vi "TagDisplayContainer.vi"(7 "Name(\"\" to use uuid)":string="UI.Exp.Template") -> ()   [LabVIEW 2020, in "CSM-TagDBDisplayContainer.lvlib"]
doc: "------------- lvcsm -------------\n[CSMStates]\nItem 0 = \"Idle\"\nItem 1 = \"CSM Documentation\"\nItem 2 = \"VI Reference\"\nItem 3 = \"Error Handler\"\nItem 4 = \"Critical Error\"\nItem 5 = \"Target Timeout Error\"\nItem 6 = \"Target Error\"\nItem 7 = \"Async Response\"\nItem 8 = \"Response\"\nItem 9 = \"Async Message Posted\"\nItem 10 = \"Initialize Core Data\"\nItem 11 = \"Exit\"\nItem 12 = \"Data: Initialize\"\nItem 13 = \"Data: Update Indicators\"\nItem 14 = \"Data: Load Attributes\"\nItem 15 = \"Data: Save Attributes\"\nItem 16 = \"Data: Cleanup\"\nItem 17 = \"Macro: Initialize\"\nItem 18 = \"Macro: Exit\"\nItem 19 = \"API: Set TagDB\"\nItem 20 = \"API: Switch\"\nItem 21 = \"API: List Views\"\nItem 22 = \"API: Set Views\"\nItem 23 = \"API: Insert View VI\"\nItem 24 = \"API: Switch2\"\nItem 25 = \"API: Start\"\nItem 26 = \"API: Stop\"\nItem 27 = \"Action: Switch Page\"\nItem 28 = \"Action: Insert New VI\"\nItem 29 = \"Action: Remove Inserted VI\"\n\n[CSMStatus]\nItem 0 = \"Error Occurred@Error Handler\"\nItem 1 = \"Action: Switch Page@API: Switch\"\nItem 2 = \"Action: Insert New VI@API: Set Views\"\nItem 3 = \"Action: Insert New VI@API: Insert View VI\"\nItem 4 = \"Action: Insert New VI@API: Switch2\""
uses:
  CSM-TagDBDisplayContainer.lvlib
  <userlib>/_NEVSTOP/Communicable State Machine(CSM)/Communicable State Machine.lvlib
  d50deaec-bb00-4691-9d91-a2e409c005f3.vi
  a2febdbb-fb03-4ba6-9898-8a5d1d02332c.vi
  <userlib>/_NEVSTOP/Communicable State Machine(CSM)/addons/Logger/CSM File Logger.lvlib
  DefaultPage.vi
  _support/ViewMgr.lvclass
  254342f9-cc88-4ec7-9cbe-7727ec765c53.vi
  <userlib>/_NEVSTOP/Communicable State Machine(CSM)/addons/INI-Static-Variable-Support/INI-Static-Variable-Support.lvlib
  <userlib>/_NEVSTOP/TagDB/TagDB.lvlib
  1aa7de20-dba2-4569-9d21-b3d571cae75a.vi
  <userlib>/_NEVSTOP/TagDB/Add-ons/RefManager/TagDB RefManager.lvlib
  f0b5f2a1-9aad-410d-9029-a536fc851335.vi
  cfd7da07-59af-4188-a865-5baa28c295fb.vi
  4ee125aa-edfd-4ba9-916e-3b81f7112f99.vi
  74c2a64d-3a13-425c-a700-8733e2dbcbf9.vi
  d4c7a5d4-b7e3-43ab-a302-e835839241e2.vi
  b2e6f326-35d8-4857-849d-4489b6e9e474.vi
  7e569b33-bc67-48db-bbe8-4478418f5bbd.vi
  <userlib>/_NEVSTOP/Communicable State Machine(CSM)/_Polymophic/CSM - Filter Duplicated Lines.vi
  <userlib>/_NEVSTOP/TagDB/Add-ons/RefManager/_Support/UISync/_Pull Controls Value to DPs(VI).vi
  <userlib>/_NEVSTOP/TagDB/Add-ons/RefManager/_Support/UISync/_Publish DP Indicators(VI).vi
panel:
  in  "Boolean":bool
  out "TagDB":refnum<k1>
  out "PageRef":refnum<vi>
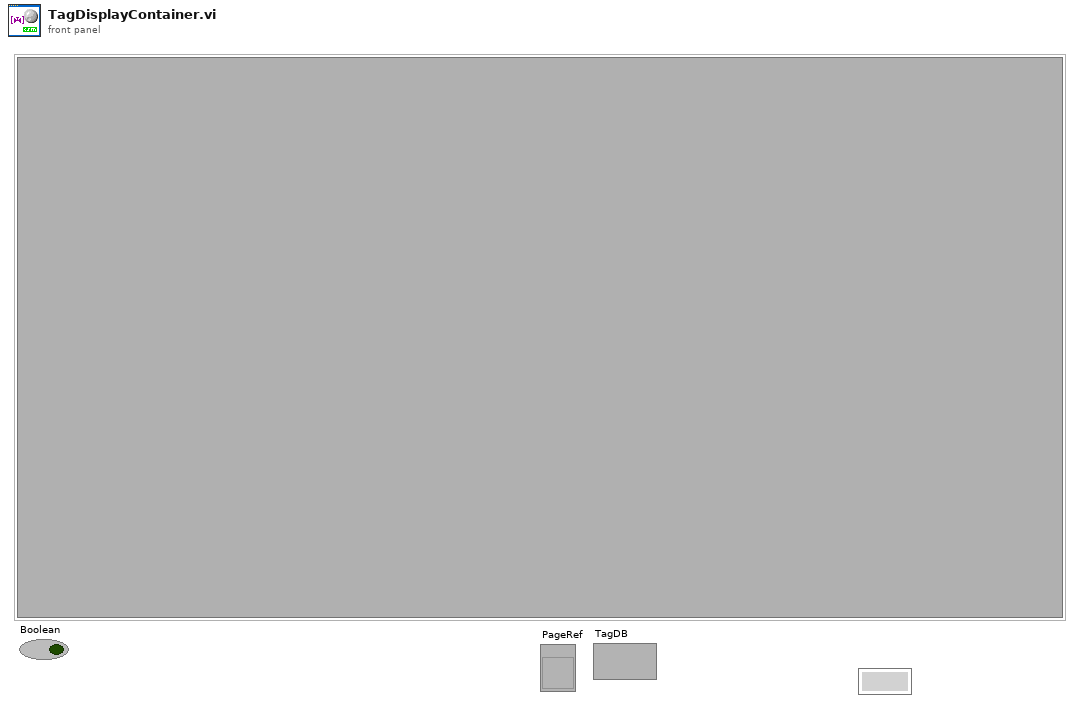
[diagram p1: front panel]
types:
  T1 = enum32{"Invalid", "Standard", "Closed", "Hidden", "Minimized", "Maximized"}
  T2 = enum32{"invalid app kind", "Development System", "Run Time System", "Student Edition", "Embedded LabVIEW", "Evaluation", "Custom"}
  T3 = cluster{"VIProto":refnum<vi>, "PageName":string}[]
  T4 = typedef "Communicable State Machine.lvlib/_CSM_Response Source Message.ctl" = cluster{"‘State":string, "’Arguments":string, "’Error":errorcluster}
  T5 = cluster{"Current VI Reference":refnum<vi>, "Close Panel on Exit?":bool}
  T6 = cluster{"Core":cluster{"Current VI Reference":refnum<vi>, "Close Panel on Exit?":bool}, "SearchingPath":path[], "PageRef":refnum<vi>, "DefaultPage":string, "PageMap":variant}
  T7 = cluster{"SearchingPath":path[], "DefaultPage":string}
  T8 = enum32{"Bad", "Idle", "Run top level", "Running"}
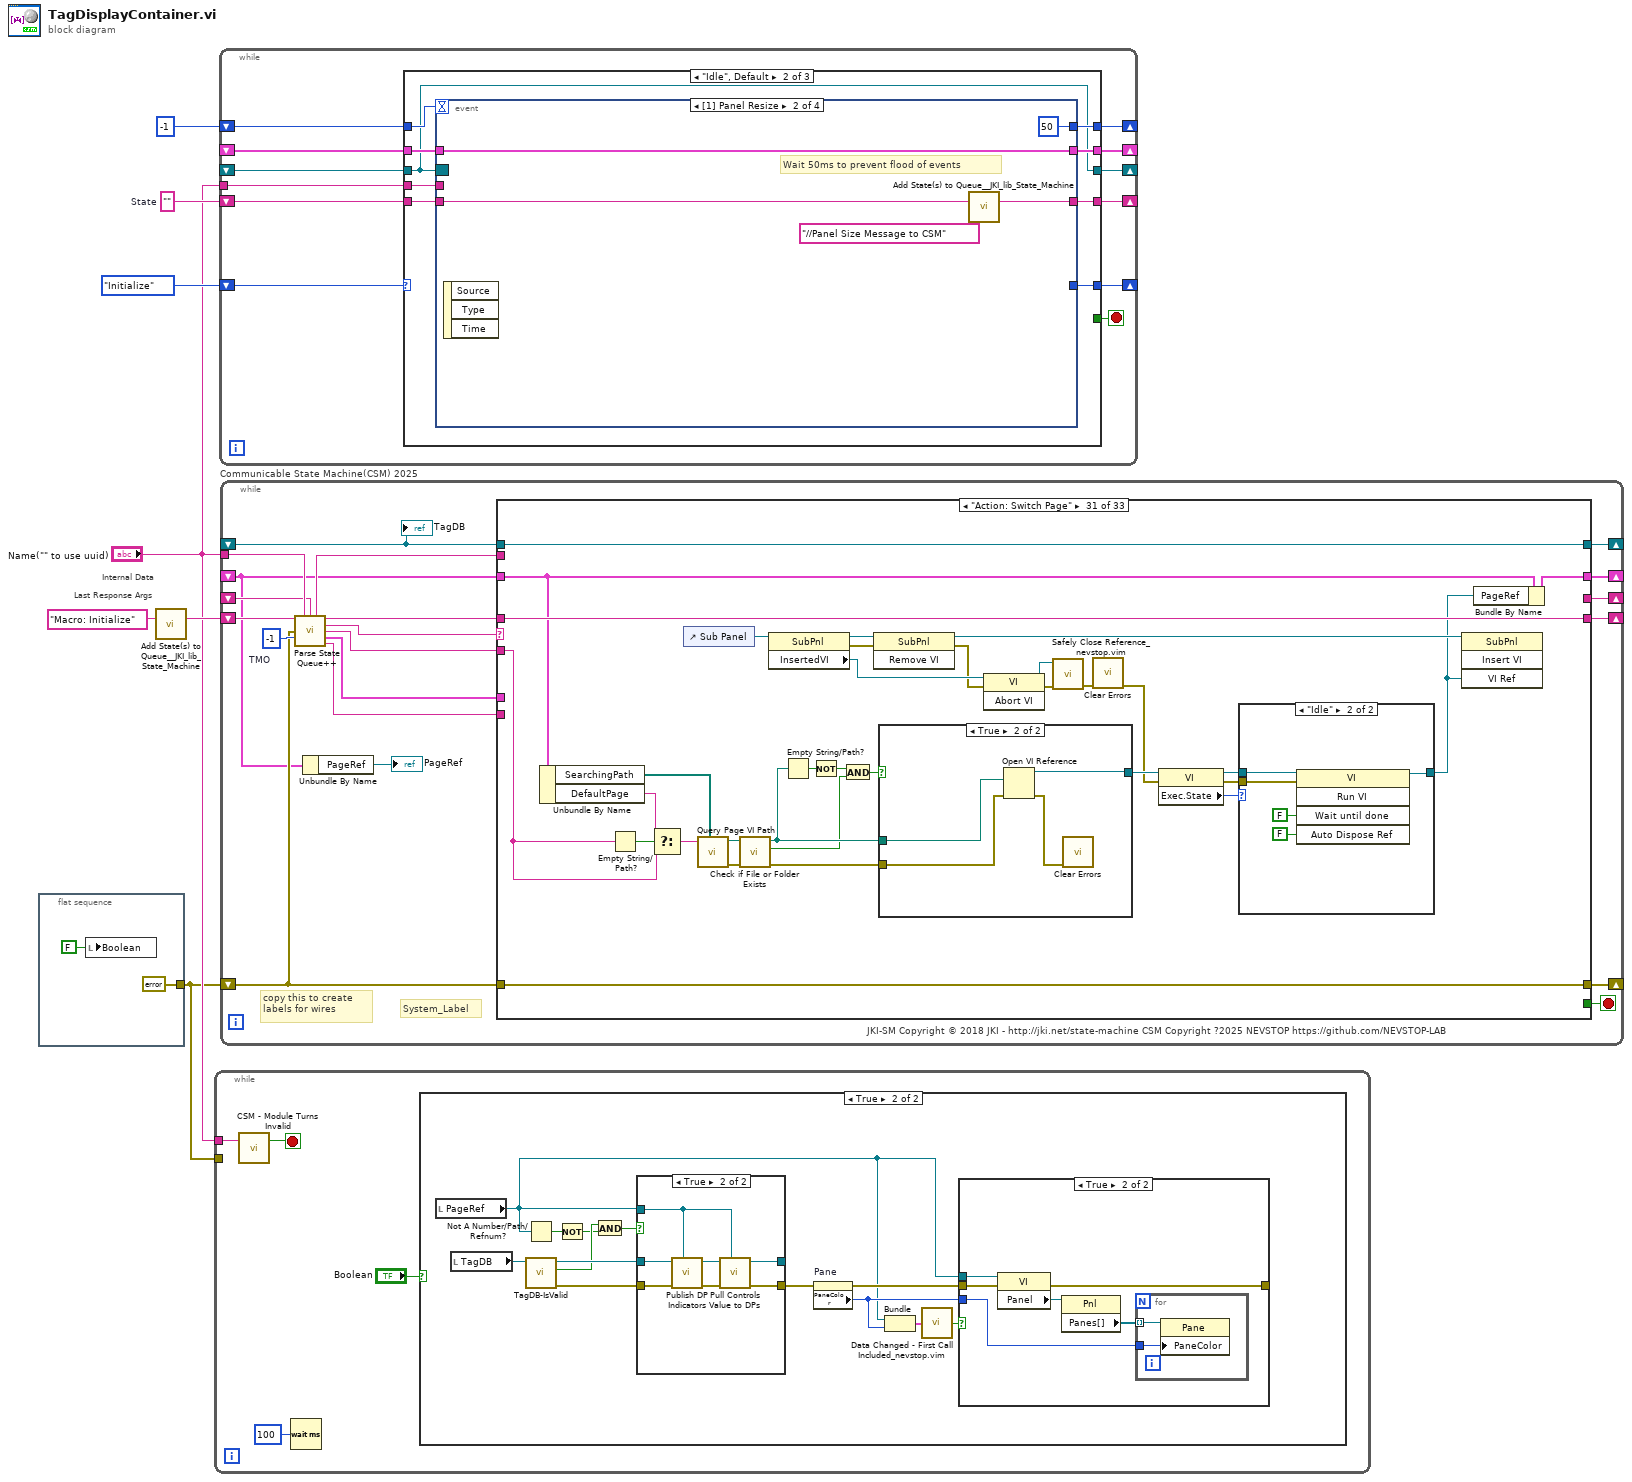
[diagram p0: block diagram]
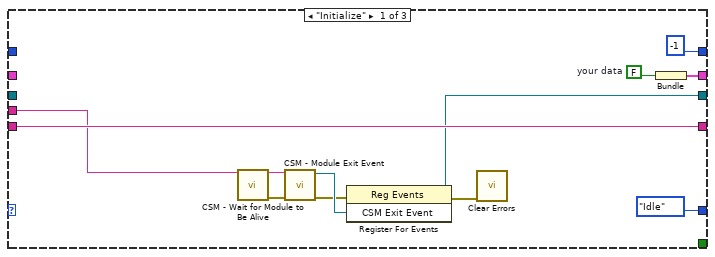
[diagram p5: hidden frame]
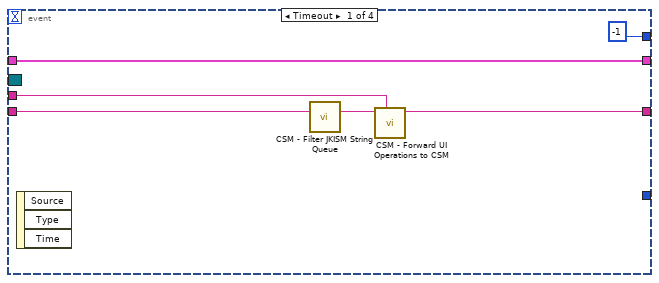
[diagram p6: hidden frame]
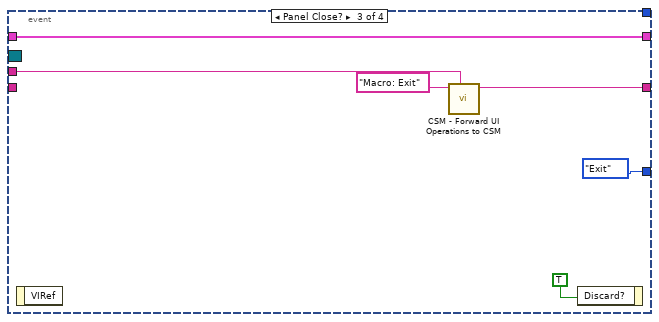
[diagram p7: hidden frame]
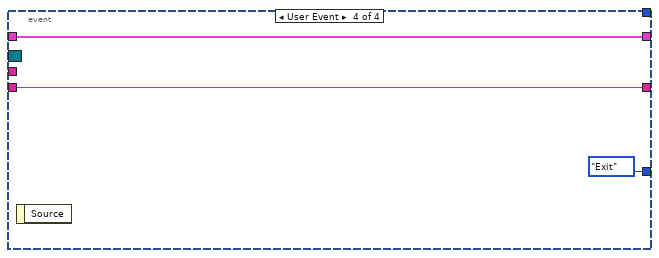
[diagram p8: hidden frame]
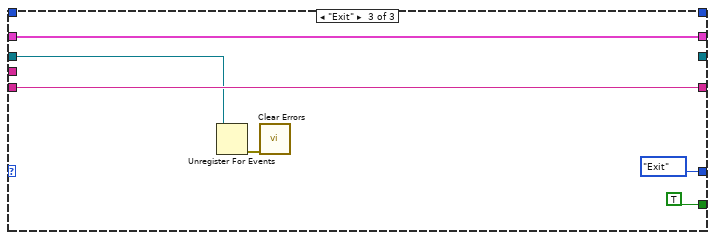
[diagram p9: hidden frame]
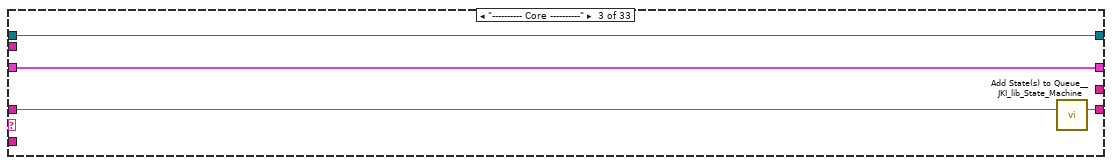
[diagram p12: hidden frame]
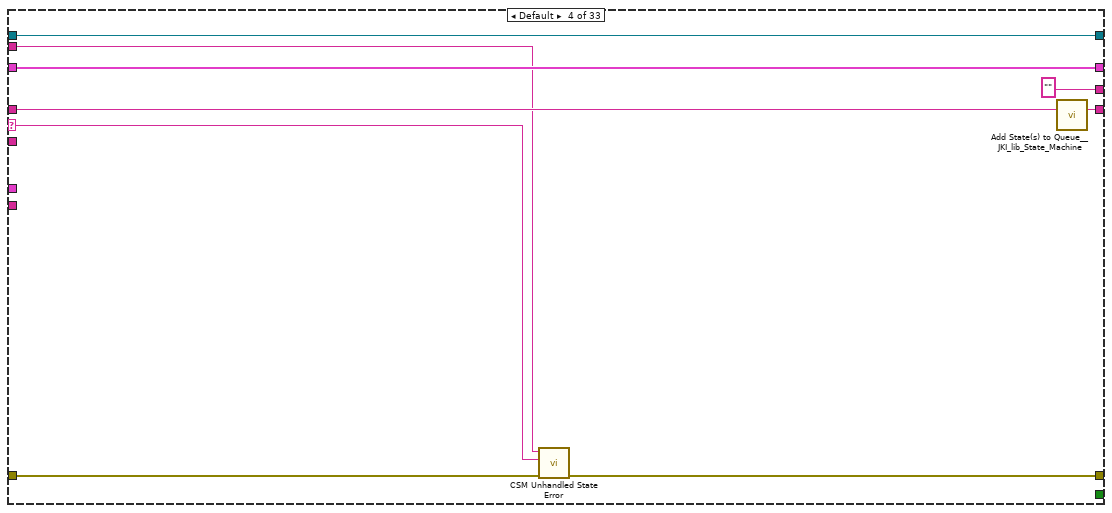
[diagram p13: hidden frame]
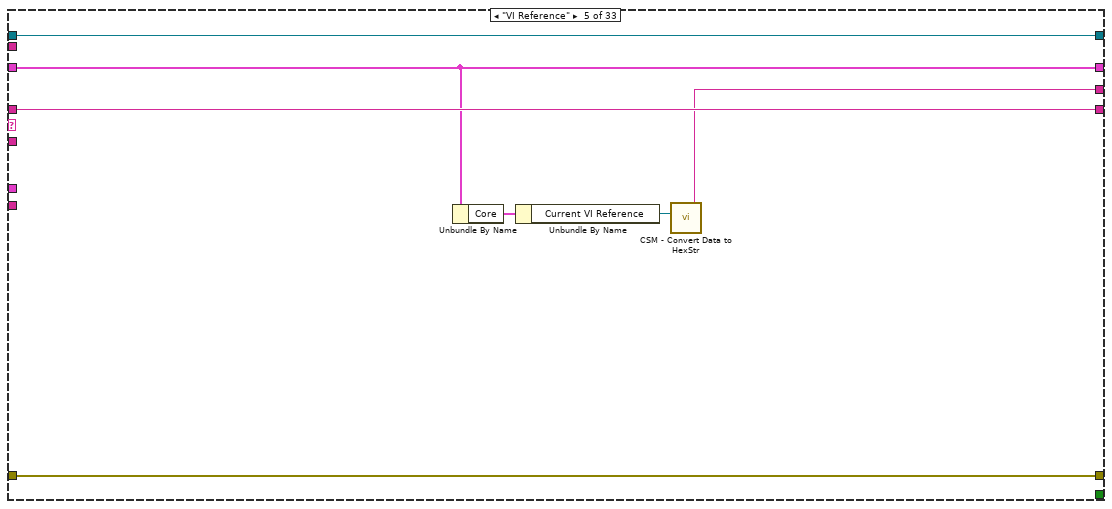
[diagram p14: hidden frame]
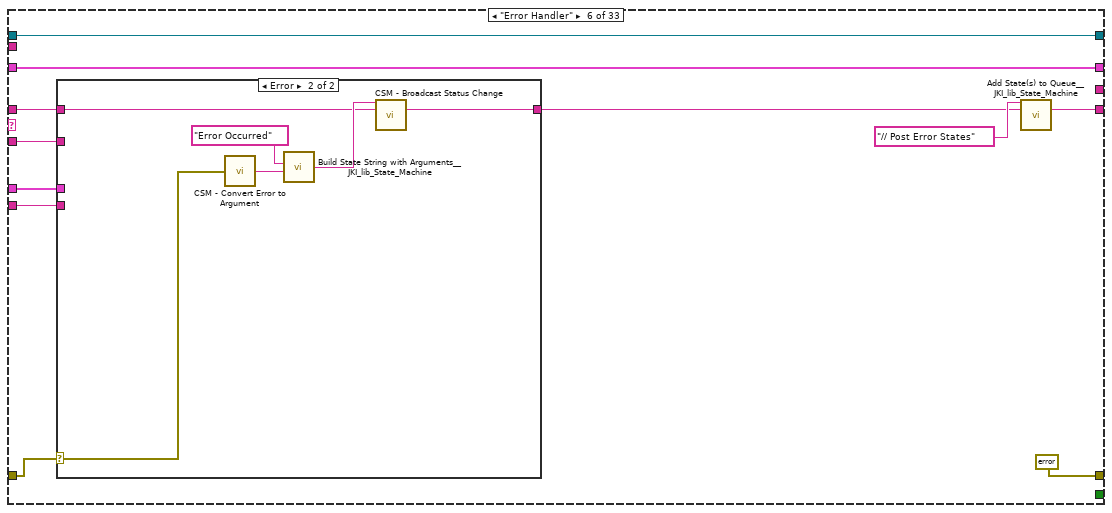
[diagram p15: hidden frame]
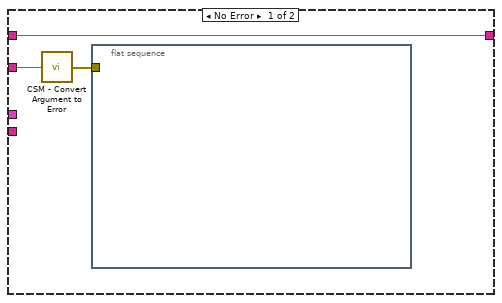
[diagram p16: hidden frame]
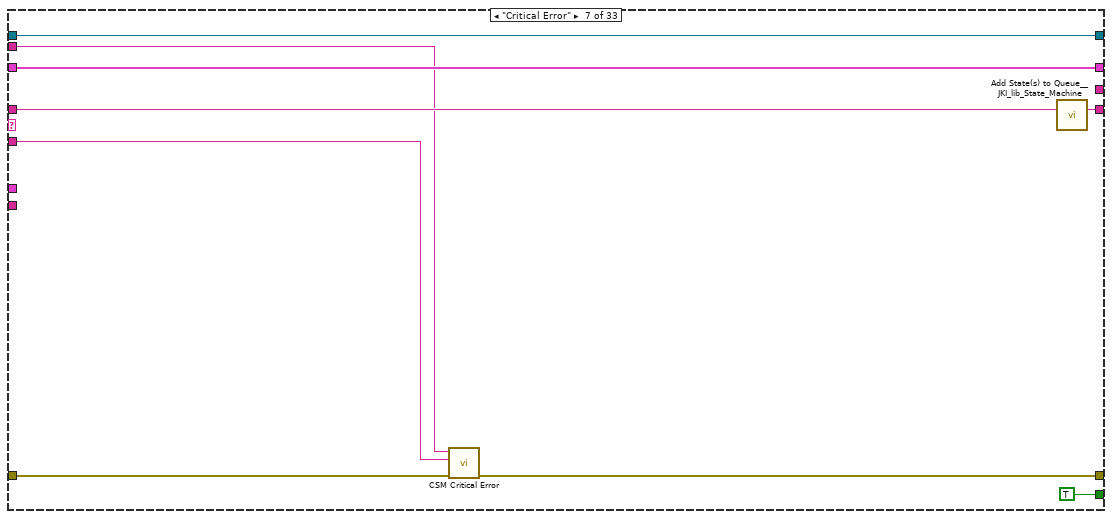
[diagram p17: hidden frame]
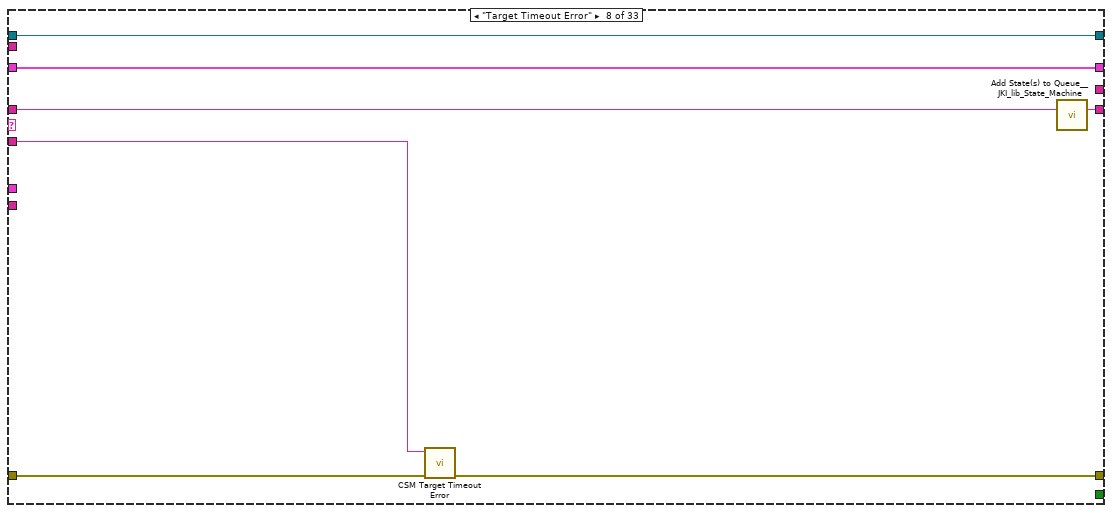
[diagram p18: hidden frame]
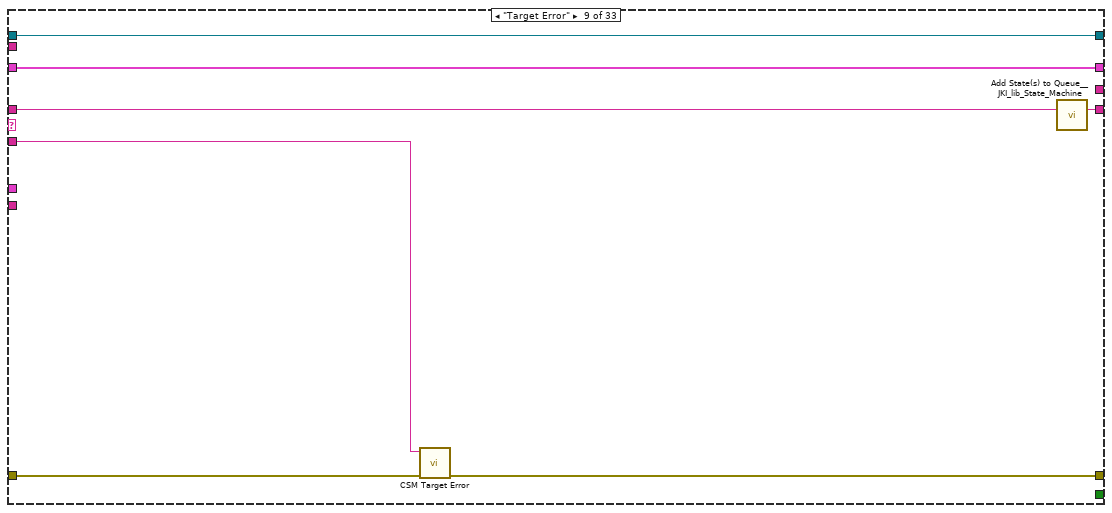
[diagram p19: hidden frame]
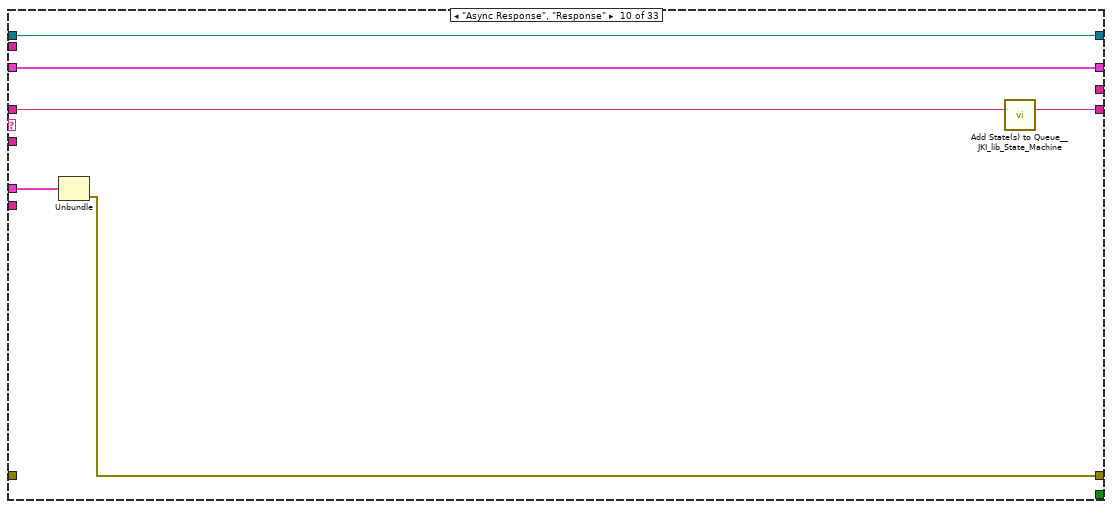
[diagram p20: hidden frame]
diagram:
  w4 = ""  # State
  # "Last Response Args"
  # "Internal Data"
  n1 = flat-sequence {
    tunnel: [errorcluster {"status"=FALSE, "code"=0, "source"=""} ("error out")] -> w1
    frame #0 {
      n2 = local write "Boolean"(FALSE ("Boolean")) -> ()
    }
  }
  n3 = call <vilib>:"Add State(s) to Queue__JKI_lib_State_Machine.vi"("State(s) in (\"\")"="Macro: Initialize" ("Init State(\"Macro: Initialize\")")) -> ("States Out"=w7:string)  [unwired: 14 in]
  n4 = while {
    tunnel: "Name(\"\" to use uuid)" -> [w12]
    tunnel: w1 -> [_]
    stop <- w13 stop-if-true
    n5 = call <userlib>:"CSM - Module Turns Invalid.vi"("CSM Name"=w12) -> ("Turn Invalid (Exit)?"=w13:bool)  [unwired: 2 in]
    n6 = Wait (ms)(milliseconds to wait=u32 100) -> ()  [unwired: 1 out]
    n7 = case shown="True" "Boolean" {
      frame False {
      }
      frame True {
        n8 = local read "PageRef"() -> (w17:refnum<vi>)
        n9 = local read "TagDB"() -> (w18:refnum<k1>)
        n10 = Not A Number/Path/Refnum?(number/path/refnum=w17) -> (NaN/Path/Refnum?=w16:bool)
        n11 = call <userlib>:"TagDB-IsValid.vi"("TagDB"=w18) -> ("error out"=w23:errorcluster, "valid TagDB?"=w24:bool, "TagDB(dup)"=w25:refnum<k1>)  [unwired: 8 in]
        n12 = Not(x=w16) -> (.not. x?=w14:bool)
        n13 = And(x=w24, y=w14) -> (x .and. y?=w15:bool)
        n14 = case shown="True" w15 {
          tunnel: w17 -> [_ w38]
          tunnel: [w37 w40] -> _
          tunnel: [w36 w39] -> w26
          tunnel: w25 -> [w37 w42]
          tunnel: w23 -> [w36 w41]
          frame False {
          }
          frame True {
            n15 = call-poly <userlib>:"Publish DP Indicators.vi"("VIRef(Caller VI)/RefMgr"=w38, "error in (no error)"=w41, "SILAPI In"=w42) -> ("error out"=w43:errorcluster, "SILAPI Out"=w44:refnum<k1>)  [unwired: 6 in, 1 out]
            n16 = call-poly <userlib>:"Pull Controls Value to DPs.vi"("VIRef(Caller VI)"=w38, "error in (no error)"=w43, "SILAPI In"=w44) -> ("error out"=w39:errorcluster, "SILAPI Out"=w40:refnum<k1>)  [unwired: 6 in, 1 out]
          }
        }
        n17 = property on="Pane" class="Pane"(error in=w26) -> (error out=w22:errorcluster, "PaneColor"=w20:u32)  [unwired: 1 in, 1 out]
        n18 = Bundle("PageRef"=w17, "PaneColor"=w20) -> (w19:cluster{"PageRef":refnum<vi>, "PaneColor":u32})  [unwired: 1 in]
        n19 = call "Data Changed - First Call Included_nevstop.vim"("Variant"=w19) -> ("Changed"=w21:bool)
        n20 = case shown="True" w21 {
          tunnel: w22 -> [w27 w33]
          tunnel: [w27 w32] -> _
          tunnel: w17 -> [_ w31]
          tunnel: w20 -> [_ w28]
          frame False {
          }
          frame True {
            n21 = property class="VI"(reference=w31, error in=w33) -> (error out=w32:errorcluster, "Panel"=w30:refnum<vi>)  [unwired: 1 out]
            n22 = property class="Pnl"(reference=w30) -> ("Panes[]"=w29:refnum<vi>[])  [unwired: 1 in, 2 out]
            n23 = for {
              tunnel: w29 -> [w35] mode=indexing
              tunnel: w28 -> [w34]
              n24 = property on="Property Node" class="Pane"(reference=w35, "PaneColor"=w34) -> ()  [unwired: 1 in, 2 out]
            }
          }
        }
      }
    }
  }
  n25 = while {
    shift-right: [w55] -> _
    shift-left: enum16{"Idle", "Initialize", "Exit"}."Initialize" -> [w56]
    tunnel: "Name(\"\" to use uuid)" -> [w53]
    shift-right: [w51] -> _
    shift-left: w4 -> [w52]
    shift-right: [w49] -> _
    shift-left: -1 -> [w50]
    shift-right: [w48] -> _
    shift-left: _ -> [w45]
    shift-right: [w47] -> _
    shift-left: _ -> [w46]
    stop <- w54 stop-if-true
    n26 = case shown="\"Idle\", Default" w56 {
      tunnel: [enum16{"Idle", "Initialize", "Exit"}."Idle" w77 enum16{"Idle", "Initialize", "Exit"}."Exit"] -> w55
      tunnel: [_ _ TRUE] -> w54
      tunnel: w53 -> [w64 w76 _]
      tunnel: w52 -> [w67 w74 w101]
      tunnel: [w67 w75 w101] -> w51
      tunnel: w50 -> [_ w72 _]
      tunnel: [-1 w73 _] -> w49
      tunnel: [w63 w69 _] -> w48
      tunnel: w45 -> [_ w69 w100]
      tunnel: [w59 w70 w98] -> w47
      tunnel: w46 -> [_ w71 w98]
      frame "Initialize" {
        w60 = FALSE  # your data
        n27 = call <userlib>:"CSM - Wait for Module to Be Alive.vi"("CSM Name"=w64) -> ("CSM Name (Dup)"=w62:string, "error out"=w61:errorcluster)  [unwired: 12 in, 1 out]
        n28 = call <userlib>:"CSM - Module Exit Event.vi"("Error In"=w61, "Name (\"\" to Use UUID) In"=w62) -> ("error out"=w57:errorcluster, "CSM Exit Event"=w65:refnum<user-event>)  [unwired: 7 in, 1 out]
        n29 = register-events(error in=w57, w65) -> (reference out=w63:refnum<event-registration>, error out=w58:errorcluster)  [unwired: 1 in]
        n30 = call <vilib>:"Clear Errors.vi"("error in (no error)"=w58) -> ()  [unwired: 5 in, 2 out]
        n31 = Bundle("your data"=w60) -> (w59:cluster{"your data":bool})  [unwired: 1 in]
      }
      frame "Idle", Default {
        n32 = event shown="[1] Panel Resize" {
          selector: w69 -> [_ _ _ _]
          dyn-events: _ -> [_ _ _ _]
          timeout: w72 -> [_ _ _ _]
          tunnel: [_ _ enum16{"Idle", "Initialize", "Exit"}."Exit" enum16{"Idle", "Initialize", "Exit"}."Exit"] -> w77
          tunnel: w76 -> [w79 _ w91 _]
          tunnel: w74 -> [w82 w88 _ w97]
          tunnel: [w80 w87 w90 w97] -> w75
          tunnel: [-1 50 _ _] -> w73
          tunnel: w71 -> [w78 w84 w89 w95]
          tunnel: [w78 w84 w89 w95] -> w70
          event Timeout {
            n33 = event-data() -> ()  [unwired: 1 in, 3 out]
            n34 = call-poly <userlib>:"CSM - Filter JKISM String Queue.vi"("States In"=w82) -> ("States Out"=w81:string)  [unwired: 14 in]
            n35 = call <userlib>:"CSM - Forward UI Operations to CSM.vi"("Name (\"\" to Use UUID)"=w79, "State(s) In (\"\")"=w81) -> ("States Out"=w80:string)  [unwired: 8 in, 1 out]
          }
          event Panel Resize {
            # "Wait 50ms to prevent flood of events"
            n36 = event-data() -> ()  [unwired: 1 in, 3 out]
            n37 = call <vilib>:"Add State(s) to Queue__JKI_lib_State_Machine.vi"("State(s) in (\"\")"=w88, "State(s) at Back (\"\")"="//Panel Size Message to CSM" ("State(s) at Back (\"\")")) -> ("States Out"=w87:string)  [unwired: 13 in]
          }
          event Panel Close? {
            n38 = event-data() -> ()  [unwired: 1 in, 1 out]
            n39 = call <userlib>:"CSM - Forward UI Operations to CSM.vi"("Name (\"\" to Use UUID)"=w91, "State(s) In (\"\")"="Macro: Exit" ("State")) -> ("States Out"=w90:string)  [unwired: 8 in, 1 out]
            n40 = event-data("Discard?"=TRUE) -> ()  [unwired: 1 in, 1 out]
          }
          event User Event {
            n41 = event-data() -> ()  [unwired: 1 in, 1 out]
          }
        }
      }
      frame "Exit" {
        n42 = Unregister For Events(event registration refnum=w100) -> (error out=w99:errorcluster)  [unwired: 1 in]
        n43 = call <vilib>:"Clear Errors.vi"("error in (no error)"=w99) -> ()  [unwired: 5 in, 2 out]
      }
    }
  }
  n44 = while "Communicable State Machine(CSM) 2025" {
    shift-right: [w118] -> _
    shift-left: _ -> [w105]
    shift-right: [w121] -> _
    shift-left: w1 -> [w108]
    shift-right: [w120] -> _
    shift-left: w7 -> [w122]
    tunnel: "Name(\"\" to use uuid)" -> [w115]
    shift-right: [w116] -> _
    shift-left: _ -> [w110]
    shift-right: [w107] -> _
    shift-left: _ -> [w106]
    stop <- w119 stop-if-true
    w117 = -1  # TMO
    # "JKI-SM Copyright © 2018 JKI - http://jki.net/state-machine CSM Copyright ?2025 NEVSTOP https://github.com/NEVSTOP-LAB"
    # "copy this to create labels for wires"
    # "System_Label"
    n45 = call <userlib>:"Parse State Queue++.vi"("State Queue"=w122, "Name (\"\" to Use UUID)"=w115, "Response Arguments"=w110, "Previous Error"=w108, "Dequeue (1 ms)"=w117) -> ("Name Used"=w109:string, "Remaining States"=w123:string, "Current State"=w111:string, "Arguments"=w112:string, "Additional Information"=w113:T4, "Source CSM"=w114:string)  [unwired: 5 in]
    n46 = Unbundle By Name(w105) -> ("PageRef"=→"PageRef":refnum<vi>)
    n47 = case shown="\"Action: Switch Page\"" w111 {
      selector: w111 -> [_ _ _ w138 _ _ _ _ _ _ _ _ _ _ _ _ _ _ _ _ _ _ _ _ _ _ _ _ _ _ _ _ _]
      tunnel: w123 -> [w125 w129 w133 w142 w148 w154 w178 w185 w192 w198 w201 w214 w219 w223 w245 w248 w263 w267 w272 w280 w283 w291 w302 w309 w314 w345 w356 w387 w393 w397 w429 w445 w494]
      tunnel: w112 -> [_ _ _ _ _ w153 w174 w182 w189 _ _ _ _ _ _ _ _ _ _ _ _ w286 w299 _ w311 w347 w352 _ _ _ w416 w443 _]
      tunnel: w105 -> [w126 w128 w131 w140 w147 w159 w176 w183 w190 w196 w200 w208 w217 w221 _ w247 w258 w265 w270 w278 w282 w290 w305 w308 w315 w350 w355 w389 w392 w395 w423 w446 w484]
      tunnel: [_ _ _ w135 w149 errorcluster {"status"=FALSE, "code"=0, "source"=""} ("error out") w171 w180 w187 w194 _ _ _ _ w231 _ w259 _ _ _ _ w287 w306 w310 w322 w351 w363 _ _ _ w430 w442 w495] -> w121
      tunnel: w108 -> [_ _ _ w136 w149 w157 w172 w181 w188 _ _ _ _ _ _ _ w260 _ _ _ _ _ w306 w310 w322 w351 w363 _ _ _ w430 _ w495]
      tunnel: [w125 w129 w132 w141 w148 w155 w177 w184 w191 w197 w201 w213 w218 w222 w244 w248 w262 w266 w271 w279 w283 w291 w303 w309 w313 w346 w353 w387 w393 w396 w429 w445 w494] -> w120
      tunnel: [_ _ _ _ _ _ TRUE _ _ _ _ _ TRUE _ _ _ _ _ _ _ _ _ _ _ _ _ _ _ _ _ _ _ _] -> w119
      tunnel: [w126 w128 w131 w140 w147 w159 w176 w183 w190 w196 w200 w212 w217 w221 w236 w247 w258 w265 w270 w278 w282 w290 w305 w308 w312 w350 w354 w389 w392 w395 w400 w444 w483] -> w118
      tunnel: w114 -> [_ _ _ _ _ w152 _ _ _ _ _ _ _ _ _ _ _ _ _ _ _ _ _ _ _ _ _ _ _ _ _ _ _]
      tunnel: w113 -> [_ _ _ _ _ w151 _ _ _ w195 _ _ _ _ _ _ _ _ _ _ _ _ _ _ _ _ _ _ _ _ _ _ _]
      tunnel: [_ _ _ "" w144 _ _ _ _ _ _ _ _ _ _ _ _ _ _ _ _ _ _ _ _ _ _ _ _ _ _ _ _] -> w116
      tunnel: w109 -> [_ _ _ w137 _ _ w173 _ _ _ _ _ _ _ w238 _ _ _ _ _ _ _ _ _ _ _ _ _ _ _ _ _ _]
      tunnel: [w124 w127 w130 w134 w143 w150 w170 w179 w186 w193 w199 w202 w215 w220 refnum<k1> refnum ("TagDB") w246 w257 w264 w268 w274 w281 w288 w304 w307 w321 w349 w362 w388 w391 w394 w428 w452 w493] -> w107
      tunnel: w106 -> [w124 w127 w130 w134 w143 w150 w170 w179 w186 w193 w199 w202 w215 w220 _ w246 w257 w264 w268 w274 w281 w289 w304 w307 w321 w349 w362 w388 w391 w394 w428 w452 w493]
      frame "", "Idle" {
      }
      frame "CSM Documentation" {
      }
      frame "---------- Core ----------" {
        n48 = call <vilib>:"Add State(s) to Queue__JKI_lib_State_Machine.vi"("State(s) in (\"\")"=w133) -> ("States Out"=w132:string)  [unwired: 14 in]
      }
      frame Default {
        n49 = call <userlib>:"CSM Unhandled State Error.vi"("error in (no error)"=w136, "Undefined State"=w138, "CSM Name"=w137) -> ("error out"=w135:errorcluster)  [unwired: 8 in]
        n50 = call <vilib>:"Add State(s) to Queue__JKI_lib_State_Machine.vi"("State(s) in (\"\")"=w142) -> ("States Out"=w141:string)  [unwired: 14 in]
      }
      frame "VI Reference" {
        n51 = Unbundle By Name(w147) -> ("Core"=w146:T5)
        n52 = Unbundle By Name(w146) -> ("Current VI Reference"=w145:refnum<vi>)
        n53 = call <userlib>:"CSM - Convert Data to HexStr.vi"("Variant"=w145) -> ("HEX String (0-9,A-F)"=w144:string)  [unwired: 8 in]
      }
      frame "Error Handler" {
        n54 = case shown="Error" w157 {
          selector: w157 -> [_ w164]
          tunnel: [w163 w166] -> w156
          tunnel: w154 -> [w163 w165]
          tunnel: w153 -> [w162 _]
          tunnel: w152 -> [_ _]
          tunnel: w151 -> [_ _]
          frame No Error {
            n55 = call <userlib>:"CSM - Convert Argument to Error.vi"("Argument"=w162) -> ("Error"=w161:errorcluster)  [unwired: 4 in]
            n56 = flat-sequence {
              tunnel: w161 -> [_]
              frame #0 {
              }
            }
          }
          frame Error {
            n57 = call <userlib>:"CSM - Convert Error to Argument.vi"("Error"=w164) -> ("Argument"=w168:string)  [unwired: 4 in]
            n58 = call <vilib>:"Build State String with Arguments__JKI_lib_State_Machine.vi"("Arguments (\"\")"=w168, "State"="Error Occurred" ("Status with Arguments")) -> ("State with Arguments"=w167:string)  [unwired: 4 in]
            n59 = call <userlib>:"CSM - Broadcast Status Change.vi"("Status With Arguments"=w167, "State Queue"=w165) -> ("Remaining States"=w166:string)  [unwired: 13 in]
          }
        }
        n60 = call <vilib>:"Add State(s) to Queue__JKI_lib_State_Machine.vi"("State(s) in Front (\"\")"="// Post Error States", "State(s) in (\"\")"=w156) -> ("States Out"=w155:string)  [unwired: 13 in]
      }
      frame "Critical Error" {
        n61 = call <userlib>:"CSM Critical Error.vi"("error in (no error)"=w172, "Arugments (As Reason)"=w174, "CSM Name"=w173) -> ("error out"=w171:errorcluster)  [unwired: 8 in]
        n62 = call <vilib>:"Add State(s) to Queue__JKI_lib_State_Machine.vi"("State(s) in (\"\")"=w178) -> ("States Out"=w177:string)  [unwired: 14 in]
      }
      frame "Target Timeout Error" {
        n63 = call <userlib>:"CSM Target Timeout Error.vi"("error in (no error)"=w181, "Arguments (As CSM Name)"=w182) -> ("error out"=w180:errorcluster)  [unwired: 9 in]
        n64 = call <vilib>:"Add State(s) to Queue__JKI_lib_State_Machine.vi"("State(s) in (\"\")"=w185) -> ("States Out"=w184:string)  [unwired: 14 in]
      }
      frame "Target Error" {
        n65 = call <userlib>:"CSM Target Error.vi"("error in (no error)"=w188, "Arguments (As CSM Name)"=w189) -> ("error out"=w187:errorcluster)  [unwired: 9 in]
        n66 = call <vilib>:"Add State(s) to Queue__JKI_lib_State_Machine.vi"("State(s) in (\"\")"=w192) -> ("States Out"=w191:string)  [unwired: 14 in]
      }
      frame "Async Response", "Response" {
        n67 = Unbundle(w195) -> ("’Error"=w194:errorcluster)  [unwired: 2 out]
        n68 = call <vilib>:"Add State(s) to Queue__JKI_lib_State_Machine.vi"("State(s) in (\"\")"=w198) -> ("States Out"=w197:string)  [unwired: 14 in]
      }
      frame "Async Message Posted" {
      }
      frame "Initialize Core Data" {
        # "originally closed?"
        # "exe?"
        # "If panel starts closed or is an EXE, then close it when we exit"
        n69 = control-ref of="Current VI Reference"() -> (w206:refnum<vi>)
        n70 = property class="VI"() -> ("FP.State"=w205:T1)  [unwired: 2 in, 2 out]
        n71 = property class="App"() -> ("App.Kind"=w211:T2)  [unwired: 2 in, 2 out]
        n72 = Equal?(x=w205, y=T1."Closed" ("Front Panel Window:State")) -> (x = y?=w203:bool)
        n73 = Equal?(x=w211, y=T2."Run Time System" ("Application:Kind")) -> (x = y?=w209:bool)
        n74 = Or(x=w203, y=w209) -> (x .or. y?=w207:bool)
        n75 = Bundle By Name(cluster=w208, "Core.Current VI Reference"=w206, "Core.Close Panel on Exit?"=w207) -> (w212:T6)
        n76 = call <vilib>:"Add State(s) to Queue__JKI_lib_State_Machine.vi"("State(s) in (\"\")"=w214) -> ("States Out"=w213:string)  [unwired: 14 in]
      }
      frame "Exit" {
        n77 = call <vilib>:"Add State(s) to Queue__JKI_lib_State_Machine.vi"("State(s) in (\"\")"=w219) -> ("States Out"=w218:string)  [unwired: 14 in]
      }
      frame "---------- Data ----------" {
        n78 = call <vilib>:"Add State(s) to Queue__JKI_lib_State_Machine.vi"("State(s) in (\"\")"=w223) -> ("States Out"=w222:string)  [unwired: 14 in]
      }
      frame "Data: Initialize" {
        w224 = variant  # PageMap
        w225 = "*"  # DefaultPage
        w235 = ""  # DefaultPage
        w240 = refnum<vi> refnum  # PageRef
        w237 = path[] []  # SearchingPath
        w242 = T5 {"Current VI Reference"=refnum, "Close Panel on Exit?"=FALSE}  # Core
        n79 = Bundle("Core"=w242, "SearchingPath"=w237, "PageRef"=w240, "DefaultPage"=w235, "PageMap"=w224) -> (w243:T6)  [unwired: 1 in]
        n80 = Bundle("SearchingPath"=w237, "DefaultPage"=w235) -> (w239:T7)  [unwired: 1 in]
        n81 = call "CSM - Read Cluster Elements From Session.vim"("Section Name (\"\" as Default)"=w238, "Cluster"=w239) -> ("error out"=w231:errorcluster, "Cluster out"=w234:T7)  [unwired: 6 in]
        n82 = Unbundle By Name(w234) -> ("SearchingPath"=w233:path[], "DefaultPage"=w232:string)
        n83 = call <userlib>:"CSM Application Directory.vi"() -> ("CSM Application Dir"=w226:path)  [unwired: 11 in]
        n84 = Current VI's Path() -> (path=w229:path)
        n85 = Build Path(base path=w226, name or relative path=w225) -> (appended path=w227:path)
        n86 = call <userlib>:"First Existing Folder in Path.vi"("Stripped Path In"=w229) -> ("Stripped Path Out"=w228:path)  [unwired: 10 in]
        n87 = Build Array (concatenate)(w233, w228, w227) -> (w230:path[])
        n88 = Bundle By Name(cluster=w243, "SearchingPath"=w230, "DefaultPage"=w232) -> (w236:T6)
        n89 = call <vilib>:"Add State(s) to Queue__JKI_lib_State_Machine.vi"("State(s) in (\"\")"=w245) -> ("States Out"=w244:string)  [unwired: 14 in]
      }
      frame "Data: Update Indicators" {
      }
      frame "Data: Cleanup" {
        n90 = Unbundle By Name(w258) -> ("Core.Current VI Reference"=w261:refnum<vi>)
        n91 = control-ref of="Sub Panel"() -> (w256:refnum<vi>)
        n92 = property class="SubPnl"(reference=w256) -> (reference out=w250:refnum<vi>, error out=w251:errorcluster, "InsertedVI"=w255:refnum<vi>)  [unwired: 1 in]
        n93 = invoke class="SubPnl" method="Remove VI"(reference=w250, error in=w251) -> (error out=w249:errorcluster)  [unwired: 1 in, 2 out]
        n94 = Close Reference(reference=w261, error in (no error)=w260) -> (error out=w259:errorcluster)
        n95 = invoke class="VI" method="Abort VI"(reference=w255, error in=w249) -> (reference out=w253:refnum<vi>, error out=w254:errorcluster)  [unwired: 1 in, 1 out]
        n96 = call "Safely Close Reference_nevstop.vim"("error in (no error)"=w254, "Reference"=w253) -> ("error out"=w252:errorcluster)  [unwired: 9 in]
        n97 = call <vilib>:"Clear Errors.vi"("error in (no error)"=w252) -> ()  [unwired: 5 in, 2 out]
        n98 = call <vilib>:"Add State(s) to Queue__JKI_lib_State_Machine.vi"("State(s) in (\"\")"=w263) -> ("States Out"=w262:string)  [unwired: 14 in]
      }
      frame "---------- Macro ----------" {
        n99 = call <vilib>:"Add State(s) to Queue__JKI_lib_State_Machine.vi"("State(s) in (\"\")"=w267) -> ("States Out"=w266:string)  [unwired: 14 in]
      }
      frame "Macro: Initialize" {
        n100 = call <vilib>:"Add State(s) to Queue__JKI_lib_State_Machine.vi"("State(s) in Front (\"\")"="Data: Initialize\nInitialize Core Data\nData: Update Indicators\nAction: Switch Page\nAPI: Start", "State(s) in (\"\")"=w272) -> ("States Out"=w271:string)  [unwired: 13 in]
      }
      frame "Macro: Exit" {
        n101 = local write "Boolean"(FALSE ("Boolean")) -> ()
        n102 = call <vilib>:"Add State(s) to Queue__JKI_lib_State_Machine.vi"("State(s) in Front (\"\")"="//Exit Sub-Modules ", "State(s) at Back (\"\")"="\nData: Cleanup\nExit") -> ("States Out"=w276:string)  [unwired: 13 in]
        n103 = call <vilib>:"Add State(s) to Queue__JKI_lib_State_Machine.vi"("State(s) in Front (\"\")"=w276, "State(s) in (\"\")"=w280) -> ("States Out"=w279:string)  [unwired: 13 in]
      }
      frame "---------- API ----------" {
      }
      frame "API: Set TagDB" {
        n104 = call <userlib>:"Is HexStr Content.vi"("Content"=w286) -> ("hexStr"=w284:string, "HexStr Content"=w285:bool)  [unwired: 9 in]
        n105 = case shown="False" w285 {
          tunnel: w289 -> [_ w298]
          tunnel: [w294 w297] -> w288
          tunnel: [w293 w296] -> w287
          tunnel: w284 -> [w292 w295]
          frame False {
            n106 = call <userlib>:"TagDB-Obtain.vi"("name (unnamed)"=w292) -> ("error out"=w293:errorcluster, "TagDB"=w294:refnum<k1>)  [unwired: 4 in, 1 out]
          }
          frame True {
            n107 = call "CSM - Convert HexStr to Data.vim"("Type"=w298, "HEX String"=w295) -> ("Error out"=w296:errorcluster, "data"=w297:refnum<k1>)  [unwired: 6 in]
          }
        }
      }
      frame "API: Switch" {
        n108 = call <vilib>:"Build State String with Arguments__JKI_lib_State_Machine.vi"("Arguments (\"\")"=w299, "State"="Action: Switch Page") -> ("State with Arguments"=w300:string)  [unwired: 4 in]
        n109 = call <vilib>:"Add State(s) to Queue__JKI_lib_State_Machine.vi"("State(s) in Front (\"\")"=w300, "State(s) in (\"\")"=w302) -> ("States Out"=w303:string)  [unwired: 13 in]
      }
      frame "API: List Views" {
      }
      frame "API: Set Views" {
        n110 = call "Convert API String Arguments to Data.vim"("Reference Type"=T3 [], "API String"=w311) -> ("Data"=w317:T3)  [unwired: 6 in, 1 out]
        n111 = in-place {
          in-place-border: w317 -> [w326]
          in-place-border: [w324] -> w316
          n112 = in-place-cluster #1(w315) -> ("PageMap"=w328:variant)
          n113 = for {
            shift-right: [w334] -> w327
            shift-left: w328 -> [w335]
            tunnel: w326 -> [w333] mode=indexing
            n114 = Unbundle By Name(w333) -> ("PageName"=w332:string, "VIProto"=w330:refnum<vi>)
            n115 = case shown="\"\"" w332 {
              selector: w332 -> [_ w342]
              tunnel: [w340 w343] -> w331
              tunnel: w330 -> [w341 w343]
              tunnel: [w337 w342] -> w329
              frame "" {
                n116 = property class="VI"(reference=w341) -> (reference out=w340:refnum<vi>, "Path"=w339:path)  [unwired: 1 in, 1 out]
                n117 = Strip Path(path=w339) -> (name=w338:string)  [unwired: 1 out]
                n118 = Match Pattern(string=w338, regular expression=".vi$" ("string")) -> (before substring=w337:string)  [unwired: 1 in, 3 out]
              }
              frame Default {
              }
            }
            n119 = Set Variant Attribute(Variant=w335, name=w329, value=w331) -> (Variant out=w334:variant)  [unwired: 1 in, 2 out]
          }
          n120 = Index Array(array=w326) -> (element=w325:cluster{"VIProto":refnum<vi>, "PageName":string})  [unwired: 1 in]
          n121 = Unbundle By Name(w325) -> ("VIProto"=w323:refnum<vi>)
          n122 = call "Convert Data To API String Arguments.vim"("Data"=w323) -> ("API String"=w324:string)  [unwired: 7 in, 1 out]
          n123 = in-place-cluster #1("PageMap"=w327) -> (w312:T6)
        }
        n124 = call <vilib>:"Build State String with Arguments__JKI_lib_State_Machine.vi"("Arguments (\"\")"=w316, "State"="Action: Insert New VI") -> ("State with Arguments"=w319:string)  [unwired: 4 in]
        n125 = call <vilib>:"Add State(s) to Queue__JKI_lib_State_Machine.vi"("State(s) in Front (\"\")"=w319, "State(s) in (\"\")"=w314) -> ("States Out"=w313:string)  [unwired: 13 in]
      }
      frame "API: Insert View VI" {
        n126 = call <vilib>:"Build State String with Arguments__JKI_lib_State_Machine.vi"("Arguments (\"\")"=w347, "State"="Action: Insert New VI") -> ("State with Arguments"=w344:string)  [unwired: 4 in]
        n127 = call <vilib>:"Add State(s) to Queue__JKI_lib_State_Machine.vi"("State(s) in Front (\"\")"=w344, "State(s) in (\"\")"=w345) -> ("States Out"=w346:string)  [unwired: 13 in]
      }
      frame "API: Switch2" {
        n128 = call "Convert API String Arguments to Data.vim"("Reference Type"="" ("PageName"), "API String"=w352) -> ("Data"=w359:string)  [unwired: 6 in, 1 out]
        n129 = in-place {
          in-place-border: w359 -> [w370]
          in-place-border: [w376] -> w357
          n130 = in-place-cluster #2(w355) -> ("PageMap"=w372:variant, "PageRef"=w374:refnum<vi>)
          n131 = Get Variant Attribute(Variant=w372) -> (duplicate Variant=w371:variant, names=w365:string[])  [unwired: 3 in, 2 out]
          n132 = To Lower Case(string=w365) -> (all lower case string=w368:string[])
          n133 = To Lower Case(string=w370) -> (all lower case string=w367:string)
          n134 = Search 1D Array(1D array=w368, element=w367) -> (index of element=w369:i32)  [unwired: 1 in]
          n135 = case shown="-1" w369 {
            selector: w369 -> [_ w385]
            tunnel: w368 -> [w379 _]
            tunnel: w367 -> [w378 _]
            tunnel: [w377 w385] -> w366
            frame -1 {
              n136 = for {
                tunnel: w379 -> [w382] mode=indexing
                tunnel: w378 -> [w384]
                tunnel: [w381] -> w377 if=w380
                i -> [w381]
                stop <- w380 stop-if-true
                n137 = Match Pattern(string=w382, regular expression=w384, offset (0)=w381) -> (offset past match=w383:i32)  [unwired: 3 out]
                n138 = Greater Or Equal To 0?(x=w383) -> (x >= 0?=w380:bool)
              }
            }
            frame Default {
            }
          }
          n139 = Index Array(array=w365, index=w366) -> (element=w364:string)
          n140 = Get Variant Attribute(Variant=w371, name=w364, default value (empty Variant)=w374) -> (duplicate Variant=w375:variant, value=w373:refnum<vi>)  [unwired: 1 in, 2 out]
          n141 = call "Convert Data To API String Arguments.vim"("Data"=w373) -> ("API String"=w376:string)  [unwired: 7 in, 1 out]
          n142 = in-place-cluster #2("PageMap"=w375, "PageRef"=w374) -> (w354:T6)
        }
        n143 = call <vilib>:"Build State String with Arguments__JKI_lib_State_Machine.vi"("Arguments (\"\")"=w357, "State"="Action: Insert New VI") -> ("State with Arguments"=w360:string)  [unwired: 4 in]
        n144 = call <vilib>:"Add State(s) to Queue__JKI_lib_State_Machine.vi"("State(s) in Front (\"\")"=w360, "State(s) in (\"\")"=w356) -> ("States Out"=w353:string)  [unwired: 13 in]
      }
      frame "API: Start" {
        n145 = local write "Boolean"(TRUE ("Boolean")) -> ()
      }
      frame "API: Stop" {
        n146 = local write "Boolean"(FALSE ("Boolean")) -> ()
      }
      frame "---------- Action ----------" {
        n147 = call <vilib>:"Add State(s) to Queue__JKI_lib_State_Machine.vi"("State(s) in (\"\")"=w397) -> ("States Out"=w396:string)  [unwired: 14 in]
      }
      frame "Action: Switch Page" {
        n148 = Unbundle By Name(w423) -> ("SearchingPath"=w422:path[], "DefaultPage"=w417:string)
        n149 = Empty String/Path?(string/path=w416) -> (empty?=w418:bool)
        n150 = Select(t=w417, s=w418, f=w416) -> (s? t:f=w415:string)
        n151 = control-ref of="Sub Panel"() -> (w403:refnum<vi>)
        n152 = call "Query Page VI Path.vi"("searching path"=w422, "page name"=w415) -> ("Error out"=w420:errorcluster, "path"=w421:path)  [unwired: 8 in]
        n153 = call <vilib>:"Check if File or Folder Exists.vi"("error in (no error)"=w420, "path"=w421) -> ("error out"=w419:errorcluster, "file or folder exists?"=w412:bool, "dup path"=w414:path)  [unwired: 7 in]
        n154 = property class="SubPnl"(reference=w403) -> (reference out=w405:refnum<vi>, error out=w406:errorcluster, "InsertedVI"=w410:refnum<vi>)  [unwired: 1 in]
        n155 = Empty String/Path?(string/path=w414) -> (empty?=w398:bool)
        n156 = Not(x=w398) -> (.not. x?=w413:bool)
        n157 = And(x=w413, y=w412) -> (x .and. y?=w411:bool)
        n158 = invoke class="SubPnl" method="Remove VI"(reference=w405, error in=w406) -> (reference out=w401:refnum<vi>, error out=w404:errorcluster)  [unwired: 1 in, 1 out]
        n159 = case shown="True" w411 {
          tunnel: [w431 w435] -> w427
          tunnel: w414 -> [_ w434]
          tunnel: w419 -> [_ w433]
          frame False {
            n160 = vi-ref "CSM-TagDBDisplayContainer.lvlib:ViewMgr.lvclass:DefaultPage.vi"() -> (w431:refnum<vi>)
          }
          frame True {
            n161 = Open VI Reference(vi path=w434, error in (no error)=w433) -> (vi reference=w435:refnum<vi>, error out=w432:errorcluster)  [unwired: 4 in]
            n162 = call <vilib>:"Clear Errors.vi"("error in (no error)"=w432) -> ()  [unwired: 5 in, 2 out]
          }
        }
        n163 = invoke class="VI" method="Abort VI"(reference=w410, error in=w404) -> (reference out=w408:refnum<vi>, error out=w409:errorcluster)  [unwired: 1 in, 1 out]
        n164 = call "Safely Close Reference_nevstop.vim"("error in (no error)"=w409, "Reference"=w408) -> ("error out"=w407:errorcluster)  [unwired: 9 in]
        n165 = call <vilib>:"Clear Errors.vi"("error in (no error)"=w407) -> ("error out"=w402:errorcluster)  [unwired: 5 in, 1 out]
        n166 = property class="VI"(reference=w427, error in=w402) -> (reference out=w426:refnum<vi>, error out=w424:errorcluster, "Exec.State"=w425:T8)
        n167 = case shown="\"Idle\"" w425 {
          tunnel: w426 -> [w436 w439]
          tunnel: [w436 w437] -> w399
          tunnel: w424 -> [_ w438]
          frame "Bad", Default {
          }
          frame "Idle" {
            n168 = invoke class="VI" method="Run VI"(reference=w439, error in=w438, "Wait until done"=FALSE ("Wait Until Done"), "Auto Dispose Ref"=FALSE ("Auto Dispose Reference")) -> (reference out=w437:refnum<vi>)  [unwired: 1 in, 4 out]
          }
        }
        n169 = invoke on="Invoke Node" class="SubPnl" method="Insert VI"(reference=w401, "VI Ref"=w399) -> ()  [unwired: 2 in, 4 out]
        n170 = Bundle By Name(cluster=w423, "PageRef"=w399) -> (w400:T6)
      }
      frame "Action: Insert New VI" {
        n171 = Unbundle By Name(w446) -> ("PageRef"=w449:refnum<vi>)
        n172 = call "Convert API String Arguments to Data.vim"("Reference Type"=refnum<vi> refnum ("VIProto"), "API String"=w443) -> ("error out"=w451:errorcluster, "Data"=w448:refnum<vi>)  [unwired: 6 in]
        n173 = Not Equal?(x=w449, y=w448) -> (x != y?=w447:bool)
        n174 = case shown="True" w447 {
          tunnel: [w453 w471] -> w444
          tunnel: [_ w466] -> w442
          tunnel: w451 -> [_ w464]
          tunnel: w446 -> [w453 w457]
          tunnel: w448 -> [_ w463]
          frame False {
          }
          frame True {
            n175 = Unbundle By Name(w457) -> ("PageRef"=w456:refnum<vi>)
            n176 = invoke class="VI" method="Run VI"(reference=w463, error in=w464, "Wait until done"=FALSE ("Wait Until Done"), "Auto Dispose Ref"=TRUE ("Auto Dispose Reference")) -> (reference out=w468:refnum<vi>, error out=w473:errorcluster)  [unwired: 1 in, 3 out]
            n177 = invoke class="VI" method="Abort VI"(reference=w456) -> (error out=w455:errorcluster)  [unwired: 2 in, 2 out]
            n178 = control-ref of="Sub Panel"() -> (w454:refnum<vi>)
            n179 = call <vilib>:"Clear Errors.vi"("error in (no error)"=w455) -> ("error out"=w460:errorcluster)  [unwired: 5 in, 1 out]
            n180 = call <vilib>:"Clear Errors.vi"("error in (no error)"=w473) -> ()  [unwired: 5 in, 2 out]
            n181 = invoke class="SubPnl" method="Remove VI"(reference=w454, error in=w460) -> (reference out=w458:refnum<vi>, error out=w459:errorcluster)  [unwired: 1 in, 1 out]
            n182 = invoke class="SubPnl" method="Insert VI"(reference=w458, error in=w459, "VI Ref"=w468) -> (reference out=w465:refnum<vi>, error out=w472:errorcluster)  [unwired: 1 in, 2 out]
            n183 = Build Array(1144 ("specific error code to clear (0: all)"), 1145 ("specific error code to clear (0: all)")) -> (w462:i32[])
            n184 = Bundle By Name(cluster=w457, "PageRef"=w468) -> (w471:T6)
            n185 = call <vilib>:"Clear Errors.vi"("error in (no error)"=w472, "specific error code to clear (0: all)"=w462) -> ("error out"=w467:errorcluster, "specific error cleared?"=w469:bool)  [unwired: 8 in]
            n186 = case shown="True" w469 {
              tunnel: w468 -> [_ w482]
              tunnel: w467 -> [w476 w480]
              tunnel: [w476 w479] -> w466
              tunnel: w465 -> [_ w477]
              frame False {
              }
              frame True {
                n187 = invoke class="VI" method="FP.Close"(reference=w482, error in=w480) -> (reference out=w478:refnum<vi>, error out=w481:errorcluster)  [unwired: 1 in, 1 out]
                n188 = invoke class="SubPnl" method="Insert VI"(reference=w477, error in=w481, "VI Ref"=w478) -> (error out=w479:errorcluster)  [unwired: 1 in, 3 out]
              }
            }
          }
        }
      }
      frame "Action: Remove Inserted VI" {
        n189 = control-ref of="Sub Panel"() -> (w485:refnum<vi>)
        n190 = Unbundle By Name(w484) -> ("PageRef"=w487:refnum<vi>)
        n191 = invoke class="SubPnl" method="Remove VI"(reference=w485) -> (error out=w491:errorcluster)  [unwired: 2 in, 2 out]
        n192 = call <vilib>:"Clear Errors.vi"("error in (no error)"=w491) -> ("error out"=w486:errorcluster)  [unwired: 5 in, 1 out]
        n193 = invoke class="VI" method="Abort VI"(reference=w487, error in=w486) -> (reference out=w489:refnum<vi>, error out=w492:errorcluster)  [unwired: 1 in, 1 out]
        n194 = call "Safely Close Reference_nevstop.vim"("error in (no error)"=w492, "Reference"=w489) -> ("error out"=w490:errorcluster)  [unwired: 9 in]
        n195 = call <vilib>:"Clear Errors.vi"("error in (no error)"=w490) -> ()  [unwired: 5 in, 2 out]
        n196 = Bundle By Name(cluster=w484, "PageRef"=refnum<vi> refnum ("InsertedVI")) -> (w483:T6)
      }
    }
    "TagDB" <- w106
  }
